vi "DetectTriggerGivenTrack.vi"(8 "error in (no error)":errorcluster, 9 "CameraFrame":i32, 10 "Track":T1, 11 "FullWormRailsTriggeredBySmallEllipseRatio in":refnum<class "FullWormRailsTriggeredBySmallEllipseRatio.lvclass">) -> (0 "error out":errorcluster, 2 "Triggered?":bool, 3 "FullWormRailsTriggeredBySmallEllipseRatio out":refnum<class "FullWormRailsTriggeredBySmallEllipseRatio.lvclass">)   [LabVIEW 2019, in "FullWormRailsTriggeredBySmallEllipseRatio.lvclass"]
uses:
  FullWormRailsTriggeredBySmallEllipseRatio.lvclass
  WormTrackCluster.ctl
  StimulusObject.lvclass
  TrackTerminationReasonEnum.ctl
  FullWormRailsTriggeredBySmallEllipseRatio.lvclass/FullWormRailsTriggeredBySmallEllipseRatio.ctl
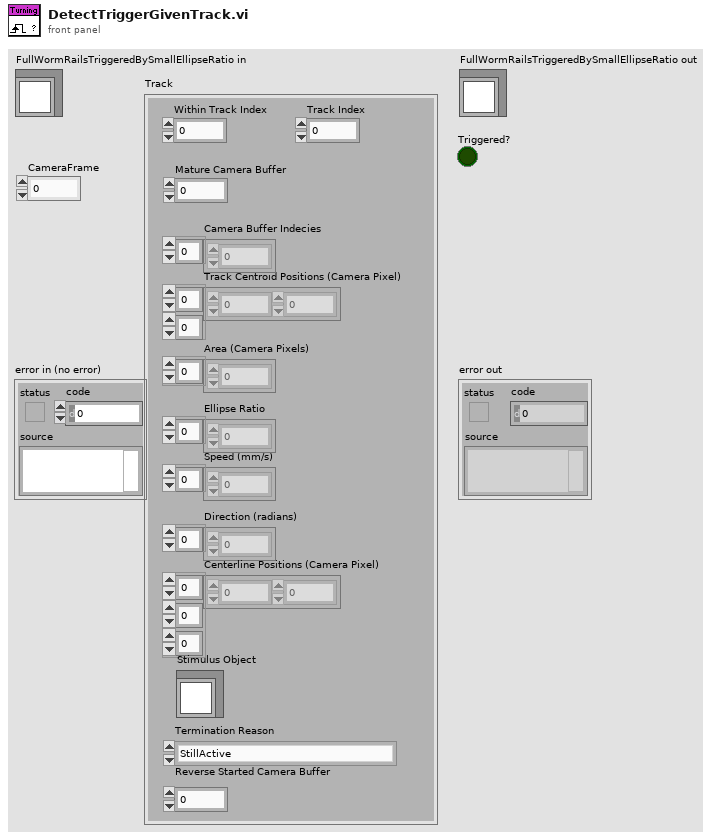
[diagram p1: front panel]
types:
  T1 = typedef "WormTrackCluster.ctl" = cluster{"Track Centroid Positions (Camera Pixel)":sgl[][], "Within Track Index":i32, "Camera Buffer Indecies":i32[], "Area (Camera Pixels)":i32[], "Speed (mm/s)":sgl[], "Direction (radians)":sgl[], "Centerline Positions (Camera Pixel)":sgl[][][], "Ellipse Ratio":sgl[], "Stimulus Object":refnum<class "StimulusObject.lvclass">, "Termination Reason":T2, "Track Index":i32, "Mature Camera Buffer":i32, "Reverse Started Camera Buffer":i32}
  T2 = typedef "TrackTerminationReasonEnum.ctl" = enum16{"StillActive", "MaxDisplacement", "NoBlobsLeft", "AreaIncrease", "AreaDecrease", "ExperimentEnded"}
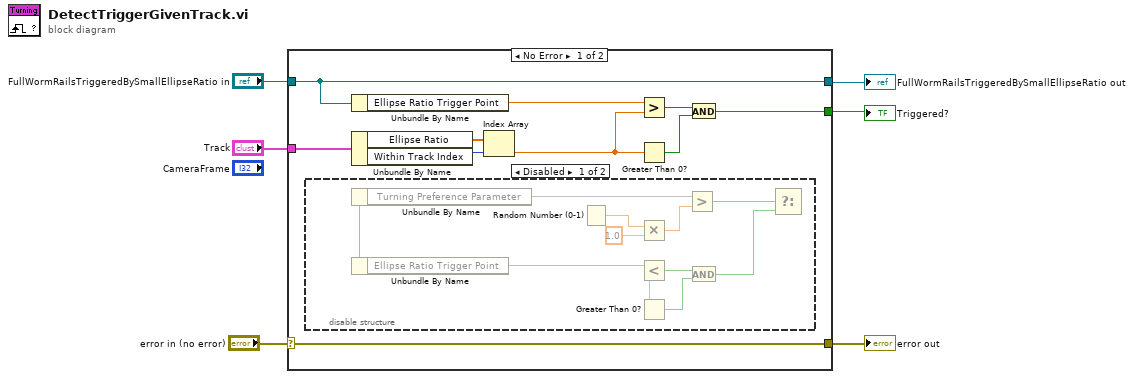
[diagram p0: block diagram]
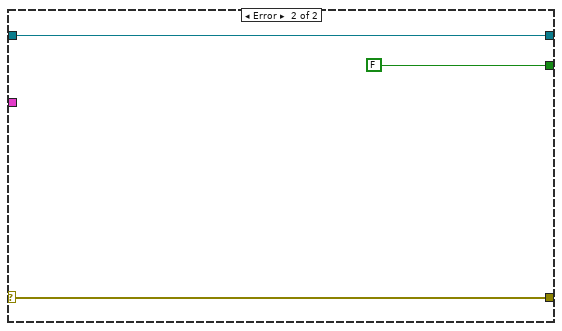
[diagram p3: hidden frame]
diagram:
  n1 = case shown="No Error" "error in (no error)" {
    selector: "error in (no error)" -> [w16 w30]
    tunnel: [w16 w30] -> w5
    tunnel: "FullWormRailsTriggeredBySmallEllipseRatio in" -> [w9 w29]
    tunnel: [w9 w29] -> w3
    tunnel: "Track" -> [w15 _]
    tunnel: [w8 FALSE] -> w1
    frame No Error {
      n2 = disable-structure shown="Disabled" {
        frame Disabled {
          n3 = Unbundle By Name() -> (w18:refnum<class "FullWormRailsTriggeredBySmallEllipseRatio.lvclass">, "Turning Preference Parameter"=w24)
          n4 = Unbundle By Name(w18) -> ("Ellipse Ratio Trigger Point"=w23)
          n5 = Random Number (0-1)() -> (number: 0 to 1=w27:dbl)
          n6 = Multiply(x=w27, y=1.0) -> (x*y=w25:dbl)
          n7 = Greater Than 0?() -> (x=w17:dbl, x > 0?=w21:bool)
          n8 = Less?(x=w23, y=w17) -> (x < y?=w22:bool)
          n9 = Greater?(x=w24, y=w25) -> (0:w20:bool)
          n10 = And(x=w22, y=w21) -> (x .and. y?=w19:bool)
          n11 = Select(s=w20, f=w19) -> ()  [unwired: 1 in, 1 out]
        }
        frame Enabled {
        }
      }
      n12 = Unbundle By Name(w9) -> ("Ellipse Ratio Trigger Point"=w12:sgl)
      n13 = Unbundle By Name(w15) -> ("Ellipse Ratio"=w14:sgl[], "Within Track Index"=w13:i32)
      n14 = Index Array(array=w14, index=w13) -> (element=w7:sgl)
      n15 = Greater?(x=w12, y=w7) -> (0:w11:bool)
      n16 = Greater Than 0?(x=w7) -> (x > 0?=w10:bool)
      n17 = And(x=w11, y=w10) -> (x .and. y?=w8:bool)
    }
    frame Error {
    }
  }
  "error out" <- w5
  "FullWormRailsTriggeredBySmallEllipseRatio out" <- w3
  "Triggered?" <- w1
